vi "打开基恩士PLC连接.vi"(8 "错误输入（无错误）":errorcluster, 10 "端号口":u16=8501, 11 "IP地址":string="192.168.0.10") -> (0 "错误输出":errorcluster, 3 "Keyence ID":refnum<k5>)   [LabVIEW 2017]
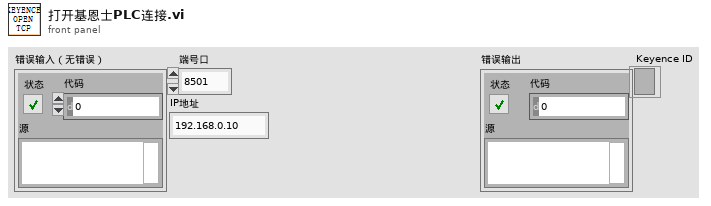
[diagram p1: front panel]
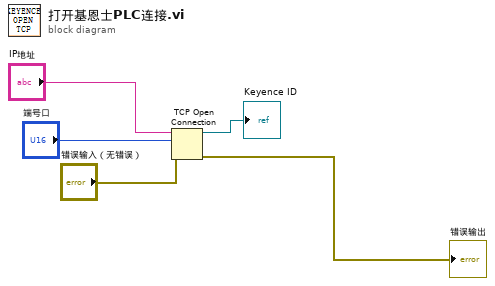
[diagram p0: block diagram]
diagram:
  n1 = TCP Open Connection(address="IP地址", remote port or service name="端号口", error in (no error)="错误输入（无错误）") -> (connection ID=→"Keyence ID":refnum<k5>, error out=→"错误输出":errorcluster)  [unwired: 2 in]
